vi "Analog Replay.vi"(5 "shift":i8=-2, 6 "memory":refnum<k21>="Replay Memory 0", 7 "settings.<user name>":T4, 8 "register bus":T1={"Speed"="Speed", "Crank Angle"="Crank Angle", "Cycle Angle"="Cycle Angle", "Crank Count"="Crank Count", "Cycle Count"="Cycle Count", "1.25 MHz Counter"="1.25 MHz Counter", "Crank Rollover"="Crank Rollover", "Cycle Rollover"="Cycle Rollover", "shared settings"={"start"=0.0, "stuck limit"=0.0}} {"shared settings"."start" format="%#.15g"}, 11 "input.<user name>":T3) -> (2 "analog value":i16)   [LabVIEW 2013, in "Engine Simulation Toolkit.lvlib" / "Analog Replay.lvlib"]
doc: "Looks up data from block memory based upon engine position and scales it based upon engine speed. This is commonly used for VR sensor simulation. \n\n<b>shift</b> - memory size is 2^N. Shift should be equal to N-16. For example if the replay memory size is 2^14 (16384 elements) then shift is equal to 14-16, -2\n<b>settings.<user name></b> - settings for the component. NI VeriStand will set these values. create a control for this input. Replace <user name> with the name you wish this component to display as inside NI VeriStand. Make this name consistent for all controls, indicators, for all VIs of this component.\n<b>input.<user name></b> - input for the component. NI VeriStand will set these values. create a control for this input. Replace <user name> with the name you wish this component to display as inside NI VeriStand. Make this name consistent for all controls, indicators, for all VIs of this component.\n<b>register bus</b> - connect this input to the output of the initialize APU VI. This contains references to APU state variables like position and speed.\n<b>memory</b> - reference to an I16 memory of size 2^N where N must be a value 10 to 16. Recommended size is 14. The memory can be set to never arbitrate to save resources. This reference should also be wired to Load Analog Replay.vi\n\n<b>analog value</b> - looked up and scaled value. Wire this to the analog output IO node."
uses:
  Analog Replay.lvlib
  Settings.ctl
  Input.ctl
  APU/Register Bus.ctl
  APU/Shared Settings.ctl
  <vilib>/Platform/TimedLoop/XDataNode/timing_clust.ctl
  <vilib>/Platform/TimedLoop/XDataNode/nitl_modes.ctl
  <vilib>/Platform/TimedLoop/XDataNode/wakeup.ctl
  <vilib>/rvi/Emulation/niFpgaSctlEmulationGetInTimedLoop.vi
  <vilib>/rvi/Emulation/niFpgaEmulationReportErrorSimple.vi
  <vilib>/rvi/Emulation/niFpgaGetClockAttributes.vi
  <vilib>/rvi/Emulation/niFpgaCriticalErrorInLSC.vi
  <vilib>/rvi/DataTransferAndStorage/Container/Common/niFpgaContainerExecOnDevCompGetState.vi
  <vilib>/rvi/DataTransferAndStorage/Register/Emulation/niFpgaRegisterEmulationFpgaImpl.vi
  <instcachedir>/0/niFpgaRegisterEmulationFpgaImpl_DCF4BC0110594B98B44A971D60CEEC4D.lvgen/niFpgaRegisterEmulationFpgaImpl_DCF4BC0110594B98B44A971D60CEEC4D_005.vi
  <vilib>/rvi/DataTransferAndStorage/Container/Common/niFpgaContainerGetUniqueNameForEmu.vi
  <instcachedir>/0/niFpgaRegisterEmulationFpgaImpl_DCF4BC0110594B98B44A971D60CEEC4D.lvgen/niFpgaRegisterEmulationFpgaImpl_DCF4BC0110594B98B44A971D60CEEC4D_006.vi
  <vilib>/rvi/Memory/Memory_Emulation/nirvimemoryFastEmulationFpgaImpl.vi
  <instcachedir>/0/nirvimemoryFastEmulationFpgaImpl_5FBAB50466BC4C939F684F8805638BFC.lvgen/nirvimemoryFastEmulationFpgaImpl_5FBAB50466BC4C939F684F8805638BFC_002.vi
  <vilib>/rvi/Memory/Memory_Emulation/niFpgaMemoryEmulationCacheClearOnFirstRun.vi
  <vilib>/rvi/Memory/Memory_Emulation/nirvimemoryEmulationManagerCache_MakeExclusive.vi
  <vilib>/rvi/Memory/Memory_Emulation/niFpgaMemoryEmulationValidateCache.vi
  <vilib>/rvi/Memory/Memory_Emulation/nirvimemoryEmulationManagerCache_ReleaseExclusive.vi
  <vilib>/rvi/Memory/Memory_Emulation/nirvimemoryEmulationManagerCache_InsertValue.vi
  <vilib>/Utility/error.llb/Clear Errors.vi
  <vilib>/rvi/Memory/Memory_Emulation/nirvimemoryEmulationManagerCache_GetValue.vi
  <vilib>/Platform/TimedLoop/XDataNode/XDataNode.xnode
  <vilib>/rvi/DataTransferAndStorage/Container/XNode/niFpgaContainer.xnode
  <vilib>/rvi/DataTransferAndStorage/Register/Emulation/niFpgaRegisterEmulationRefIn.vi
  <vilib>/rvi/Memory/Memory_Emulation/niFpgaMemoryEmulationRefIn.vi
  <vilib>/Platform/TimedLoop/XDataNode/XDNodeRunTimeDep.lvlib
  APU/APU.lvlib
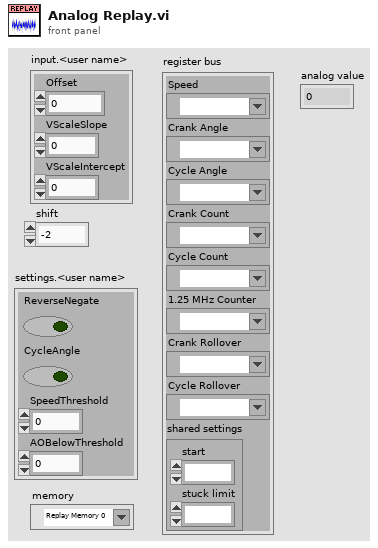
[diagram p1: front panel]
types:
  T1 = typedef "Engine Simulation Toolkit.lvlib/APU.lvlib/Register Bus.ctl" = cluster{"Speed":refnum<k21>, "Crank Angle":refnum<k21>, "Cycle Angle":refnum<k21>, "Crank Count":refnum<k21>, "Cycle Count":refnum<k21>, "1.25 MHz Counter":refnum<k21>, "Crank Rollover":refnum<k21>, "Cycle Rollover":refnum<k21>, "shared settings":T2}
  T2 = typedef "Engine Simulation Toolkit.lvlib/APU.lvlib/Shared Settings.ctl" = cluster{"start":fxp<+,17,17>, "stuck limit":fxp<+,18,18>}
  T3 = typedef "Engine Simulation Toolkit.lvlib/Analog Replay.lvlib/Input.ctl" = cluster{"Offset":i16, "VScaleSlope":fxp<+,18,6>, "VScaleIntercept":fxp<+/-,18,3>}
  T4 = typedef "Engine Simulation Toolkit.lvlib/Analog Replay.lvlib/Settings.ctl" = cluster{"ReverseNegate":bool, "CycleAngle":bool, "SpeedThreshold":fxp<+/-,23,2>, "AOBelowThreshold":i16}
  T5 = typedef "XDNodeRunTimeDep.lvlib/timing_clust.ctl" = cluster{"Expected End [f-1]":u64, "Actual End [f-1]":u64, "Finished Late? [f-1]":bool, "Expected End [i-1]":u64, "Actual End [i-1]":u64, "Finished Late? [i-1]":bool, "Expected Start [i]":u64, "Actual Start [i]":u64, "Expected Start [f]":u64, "Actual Start [f]":u64, "Source Name":string, "Structure Name":string, "Period":i64, "Deadline":i64, "Offset":i64, "Start":i64, "Priority":i32, "Timeout":i32, "Mode":T6, "Wakeup Reason":T7, "Error":errorcluster, "Source Type":string, "Secondary Source Type":string, "Global End Time":u64, "Global Start Time":u64, "Frame Duration":u64, "Iteration Duration":u64, "Assigned CPU":i32, "I/O Scan Engine Mode":u32}
  T6 = typedef "XDNodeRunTimeDep.lvlib/nitl_modes.ctl" = enum32{"No Change", "Process missed periods, maintain original phase", "Discard missed periods, maintain original phase", "Process missed periods, ignore original phase", "Discard missed periods, ignore original phase"}
  T7 = typedef "XDNodeRunTimeDep.lvlib/wakeup.ctl" = enum32{"Normal", "Aborted", "Asynchronous wakeup", "Timing source error", "Timed loop error", "Timeout"}
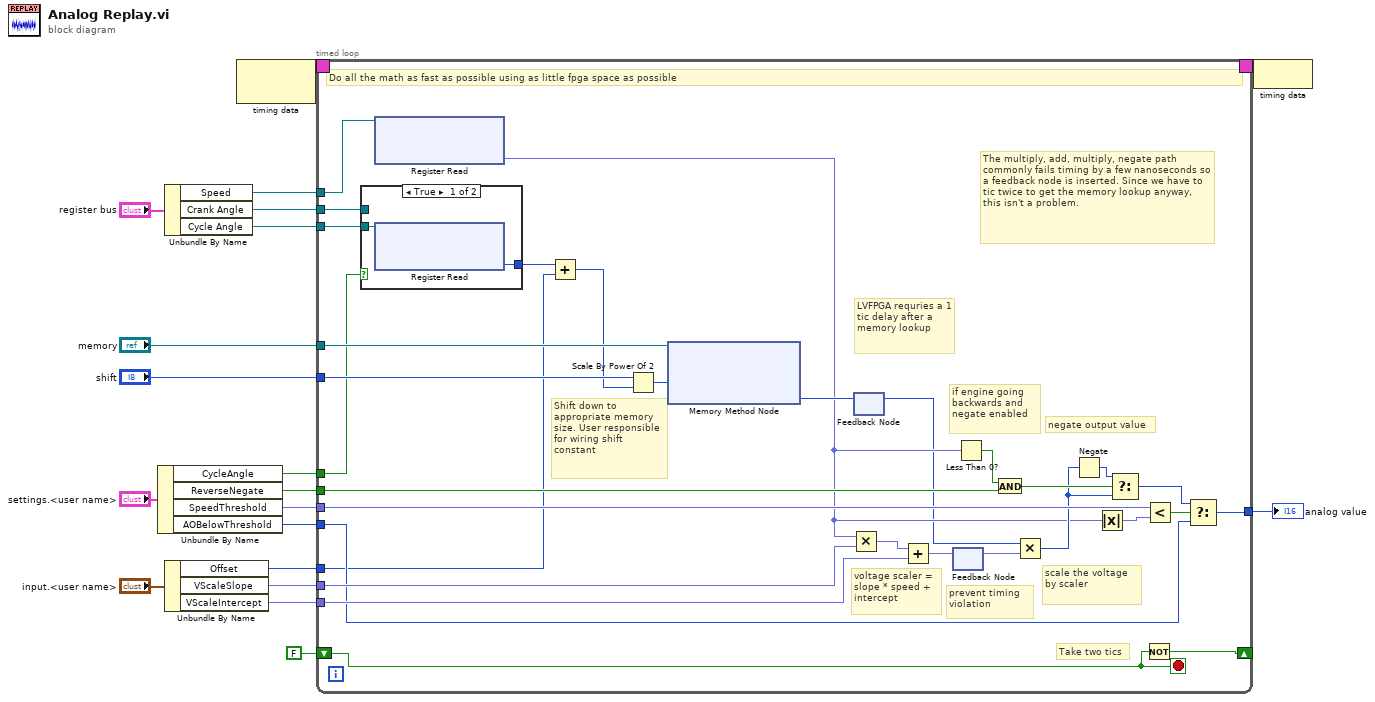
[diagram p0: block diagram]
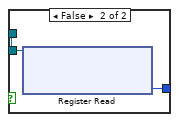
[diagram p2: hidden frame]
diagram:
  n1 = Unbundle By Name("settings.<user name>") -> ("CycleAngle"=w5:bool, "ReverseNegate"=w10:bool, "SpeedThreshold"=w7:fxp<+/-,23,2>, "AOBelowThreshold"=w6:i16)
  n2 = Unbundle By Name("register bus") -> ("Speed"=w11:refnum<k21>, "Crank Angle"=w12:refnum<k21>, "Cycle Angle"=w13:refnum<k21>)
  n3 = Unbundle By Name("input.<user name>") -> ("Offset"=w4:i16, "VScaleSlope"=w9:fxp<+,18,6>, "VScaleIntercept"=w8:fxp<+/-,18,3>)
  n4 = node-c288() -> (w3:T5)  [unwired: 1 in]
  n5 = timed-loop {
    timing: w3 -> [_]
    timing-out: [_] -> w2
    tunnel: "shift" -> [w50]
    tunnel: "memory" -> [w49]
    tunnel: [w48] -> w14
    tunnel: w13 -> [w47]
    tunnel: w12 -> [w46]
    tunnel: w11 -> [w45]
    tunnel: w10 -> [w44]
    tunnel: w9 -> [w43]
    tunnel: w8 -> [w42]
    tunnel: w7 -> [w41]
    tunnel: w6 -> [w40]
    tunnel: w5 -> [w39]
    tunnel: w4 -> [w38]
    shift-right: [w22] -> _
    shift-left: FALSE -> [w23]
    stop <- w23 stop-if-true
    # "Shift down to appropriate memory size. User responsible for wiring shift constant"
    # "The multiply, add, multiply, negate path commonly fails timing by a few nanoseconds so a feedback node is inserted. Since we have to tic twice to get the memory lookup anyway, this isn't a problem."
    # "prevent timing violation"
    # "Take two tics"
    # "LVFPGA requries a 1 tic delay after a memory lookup"
    # "negate output value"
    # "if engine going backwards and negate enabled"
    # "scale the voltage by scaler"
    # "voltage scaler = slope * speed + intercept"
    # "Do all the math as fast as possible using as little fpga space as possible"
    n6 = case shown="True" w39 {
      tunnel: w47 -> [w52 _]
      tunnel: w46 -> [_ w54]
      tunnel: [w51 w53] -> w27
      frame True {
        n7 = xnode ("Register Read")("Register In"=w52) -> ("Data"=w51:u16)  [unwired: 1 out]
      }
      frame False {
        n8 = xnode ("Register Read")("Register In"=w54) -> ("Data"=w53:u16)  [unwired: 1 out]
      }
    }
    n9 = xnode ("Register Read")("Register In"=w45) -> ("Data"=w31:fxp<+/-,23,2>)  [unwired: 1 out]
    n10 = Add(x=w27, y=w38) -> (x+y=w25:u16)
    n11 = Scale By Power Of 2(n=w50, x=w25) -> (x*2^n=w26:u16)
    n12 = xnode ("Memory Method Node")("Address"=w26, "Memory In"=w49) -> ("Data"=w34:i16)  [unwired: 1 out]
    n13 = Multiply(x=w31, y=w43) -> (x*y=w35:fxp<+/-,25,5>)
    n14 = feedback #1() -> (w24:i16)  [unwired: 1 in]
    n15 = feedback-in #1(w34) -> ()
    n16 = Add(x=w35, y=w42) -> (x+y=w21:fxp<+/-,25,1>)
    n17 = feedback #2() -> (w20:fxp<+/-,25,1>)  [unwired: 1 in]
    n18 = feedback-in #2(w21) -> ()
    n19 = Less Than 0?(x=w31) -> (x < 0?=w37:bool)
    n20 = And(x=w37, y=w44) -> (x .and. y?=w36:bool)
    n21 = Multiply(x=w24, y=w20) -> (x*y=w32:i16)
    n22 = Negate(x=w32) -> (-x=w33:i16)
    n23 = Absolute Value(x=w31) -> (abs(x)=w30:fxp<+,23,2>)
    n24 = Select(t=w33, s=w36, f=w32) -> (s? t:f=w28:i16)
    n25 = Not(x=w23) -> (.not. x?=w22:bool)
    n26 = Less?(x=w41, y=w30) -> (x < y?=w29:bool)
    n27 = Select(t=w28, s=w29, f=w40) -> (s? t:f=w48:i16)
  }
  "analog value" <- w14
  n28 = node-c288(w2) -> ()
